vi "evo irimager usb init.vi"(11 "xml_config":string) -> (0 "h out":i32, 1 "w out":i32, 2 "formatsdef":string, 3 "function return 2":i32)   [LabVIEW 2025, in "libirimager_direct_binding.lvlib"]
doc: "DIRECT_API int evo_irimager_usb_init(const char* xml_config);"
uses:
  libirimager_direct_binding.lvlib
  libirimager.dll
panel:
  out "xml":string
  out "log":string
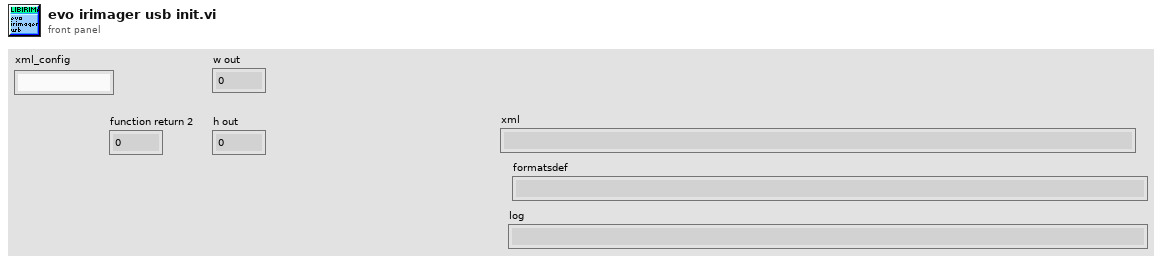
[diagram p1: front panel]
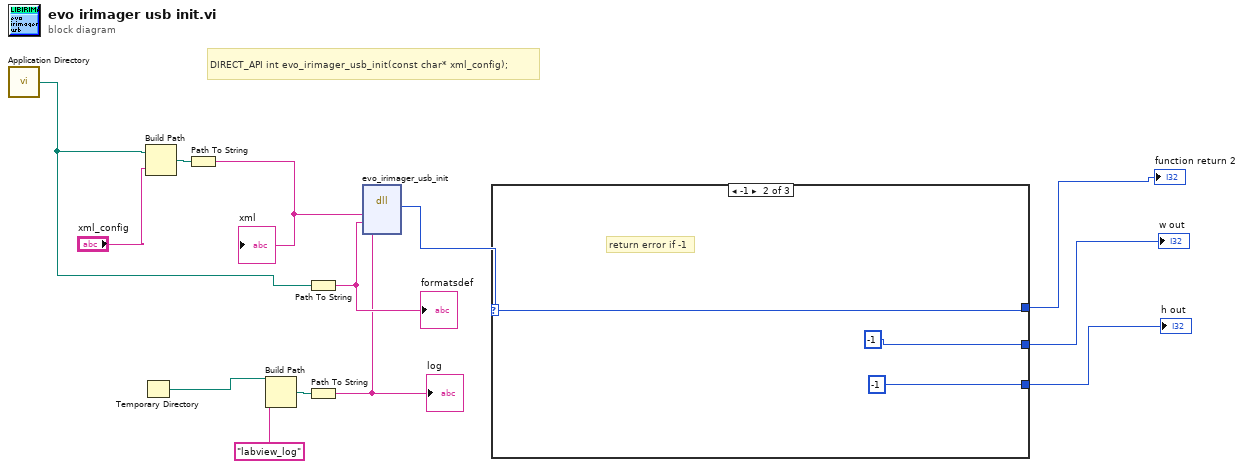
[diagram p0: block diagram]
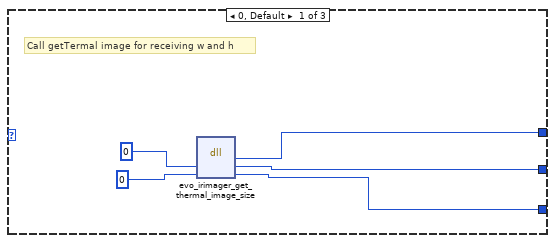
[diagram p2: hidden frame]
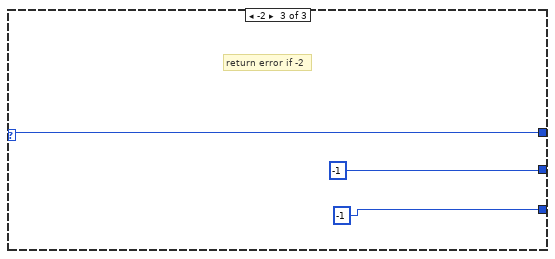
[diagram p3: hidden frame]
diagram:
  # "DIRECT_API int evo_irimager_usb_init(const char* xml_config);"
  n1 = call <vilib>:"Application Directory.vi"() -> ("Application Directory"=w3:path)
  n2 = Temporary Directory() -> (w1:path)
  n3 = Build Path(base path=w3, name or relative path="xml_config") -> (appended path=w5:path)
  n4 = Path To String(path=w5) -> (string=w4:string)
  "xml" <- w4
  n5 = Build Path(base path=w1, name or relative path="labview_log" ("String")) -> (appended path=w7:path)
  n6 = Path To String(path=w3) -> (string=w9:string)
  "formatsdef" <- w9
  n7 = Path To String(path=w7) -> (string=w6:string)
  "log" <- w6
  n8 = dll-call lib="C:/Users/mayhe/OneDrive/Documents/GitHub/In-situ-monitoring-of-powder-bed-fusion-additive-manufacturing/system_development/Orichalcum/v0.2/Software_design/thermal-camera/VI/libirimager.dll" fn="evo_irimager_usb_init"("xml_config"=w4, "formats_def"=w9, "log_file"=w6) -> ("Rückgabetyp"=w10:i32)  [unwired: 6 in, 2 out]
  n9 = case shown="-1" w10 {
    selector: w10 -> [_ w21 w24]
    tunnel: [w17 -1 -1] -> w13
    tunnel: [w16 -1 -1] -> w12
    tunnel: [w18 w21 w24] -> w11
    frame 0, Default {
      # "Call getTermal image for receiving w and h"
      n10 = dll-call lib="C:/Users/mayhe/OneDrive/Documents/GitHub/In-situ-monitoring-of-powder-bed-fusion-additive-manufacturing/system_development/Orichalcum/v0.2/Software_design/thermal-camera/VI/libirimager.dll" fn="evo_irimager_get_thermal_image_size"("w"=0, "h"=0) -> ("Rückgabetyp"=w18:i32, "w"=w17:i32, "h"=w16:i32)  [unwired: 3 in, 2 out]
    }
    frame -1 {
      # "return error if -1"
    }
    frame -2 {
      # "return error if -2"
    }
  }
  "function return 2" <- w11
  "w out" <- w13
  "h out" <- w12
